vi "Get gRPC Device Server Location.vi"(8 "error in":errorcluster, 10 "session name":string, 11 "instrument in":refnum<class "ISession Factory.lvclass">) -> (0 "error out":errorcluster, 1 "using device service":bool, 2 "remote connection options":T1, 3 "instrument out":refnum<class "ISession Factory.lvclass">, 4 "location unique id":u64)   [LabVIEW 2020, in "Plug-In SDK Session Management V1 API.lvlib" / "Session Reservation.lvclass"]
uses:
  Session Reservation.lvclass
  Sessions/Instrument Sessions/ISession Factory/ISession Factory.lvclass
  Sessions/Instrument Sessions/ISession Factory/Remote Connection Options.ctl
  Discovery V1/TypeDefs/Service Location FGV Action.ctl
  gRPC/Generated APIs/ni/measurementlink/discovery/v1/RPC Messages/ni_measurementlink_discovery_v1_ResolveServiceRequest.ctl
  Discovery V1/Plug-In SDK Discovery V1 API.lvlib
  gRPC/Generated APIs/ni/measurementlink/discovery/v1/ni.measurementlink.discovery.v1.lvlib
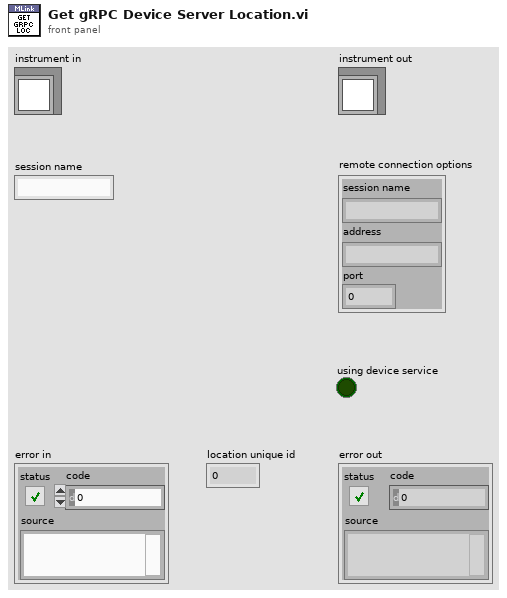
[diagram p1: front panel]
types:
  T1 = typedef "Plug-In SDK Instrument Sessions.lvlib/ISession Factory.lvclass/Remote Connection Options.ctl" = cluster{"session name":string, "address":string, "port":u32}
  T2 = typedef "ni.measurementlink.discovery.v1.lvlib/ni_measurementlink_discovery_v1_ResolveServiceRequest.ctl" = cluster{"provided_interface":string, "service_class":string}
  T3 = typedef "Plug-In SDK Discovery V1 API.lvlib/Service Location FGV Action.ctl" = enum16{"Get Service Location", "Reresolve Service Location"}
  T4 = typedef "ni.measurementlink.discovery.v1.lvlib/ni_measurementlink_discovery_v1_ServiceLocation.ctl" = cluster{"location":string, "insecure_port":string, "ssl_authenticated_port":string}
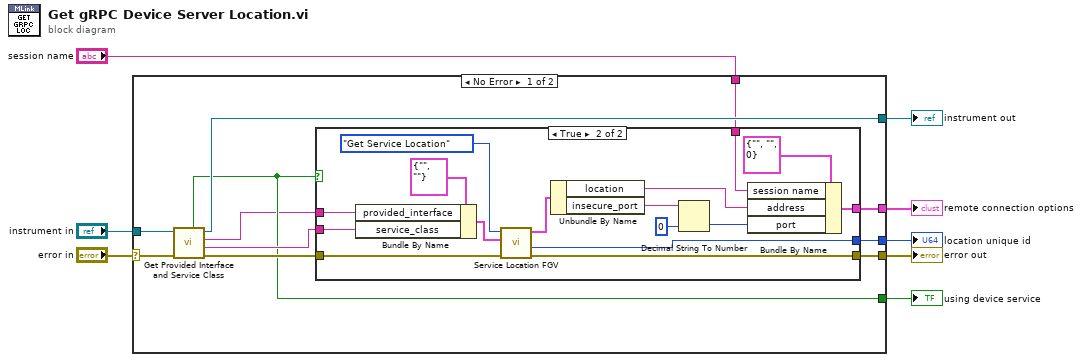
[diagram p0: block diagram]
diagram:
  n1 = case shown="No Error" "error in" {
    selector: "error in" -> [w15 w38]
    tunnel: [w19 w38] -> w8
    tunnel: [w18 w37] -> w7
    tunnel: "instrument in" -> [w16 w37]
    tunnel: [w14 _] -> w4
    tunnel: "session name" -> [w13 _]
    tunnel: [w11 _] -> w2
    tunnel: [w10 _] -> w1
    frame No Error {
      n2 = call "Get Provided Interface and Service Class.vi"("error in"=w15, "instrument in"=w16) -> ("error out"=w17:errorcluster, "service class"=w12:string, "provided interface"=w9:string, "instrument out"=w18:refnum<class "ISession Factory.lvclass">, "using device service"=w11:bool)  [unwired: 5 in]
      n3 = case shown="True" w11 {
        tunnel: [w20 w33] -> w19
        tunnel: w12 -> [_ w32]
        tunnel: w9 -> [_ w31]
        tunnel: w17 -> [w20 w27]
        tunnel: [_ w23] -> w14
        tunnel: w13 -> [_ w22]
        tunnel: [_ w21] -> w10
        frame False {
        }
        frame True {
          n4 = Bundle By Name(cluster=T2 {"provided_interface"="", "service_class"=""} ("Resolve Service Request"), "provided_interface"=w31, "service_class"=w32) -> (w28:T2)
          n5 = call "Service Location FGV.vi"("error in"=w27, "resolve service request"=w28, "action"=Service_Location_FGV_Action."Get Service Location" ("Action")) -> ("error out"=w33:errorcluster, "location unique id out"=w21:u64, "service location"=w35:T4)  [unwired: 6 in]
          n6 = Unbundle By Name(w35) -> ("location"=w25:string, "insecure_port"=w34:string)
          n7 = Decimal String To Number(string=w34, default (0L)=u32 0 ("default (0 I32)")) -> (number=w24:u32)  [unwired: 1 in, 1 out]
          n8 = Bundle By Name(cluster=T1 {"session name"="", "address"="", "port"=0} ("remote connection options"), "session name"=w22, "address"=w25, "port"=w24) -> (w23:T1)
        }
      }
    }
    frame Error {
    }
  }
  "error out" <- w8
  "instrument out" <- w7
  "remote connection options" <- w4
  "using device service" <- w2
  "location unique id" <- w1
